vi "QUE.vi"(2 "C":dbl, 3 "B":dbl, 4 "A":dbl) -> (0 "x2":dbl, 1 "x1":dbl)   [LabVIEW 2017]
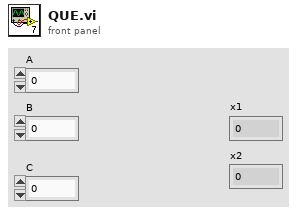
[diagram p1: front panel]
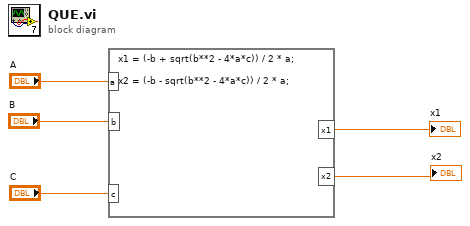
[diagram p0: block diagram]
diagram:
  n1 = formula code="x1 = (-b + sqrt(b**2 - 4*a*c)) / 2 * a; \n\nx2 = (-b - sqrt(b**2 - 4*a*c)) / 2 * a;"("a"="A", "b"="B", "c"="C") -> ("x1"=→"x1":dbl, "x2"=→"x2":dbl)
